vi "AB_API Add Source Item To Array.vi"(8 "error in (no error)":errorcluster, 9 "source item ID":string, 10 "buildObject":T1, 11 "source items in":refnum<class "AB_Source.lvclass">[](array[class])) -> (0 "error out":errorcluster, 1 "index":i32, 2 "added?":bool, 3 "source items out":refnum<class "AB_Source.lvclass">[](array[class]))   [LabVIEW 2020]
uses:
  <vilib>/AppBuilder/AB_Classes/Source/AB_Source.lvclass
  <resource>/Framework/Providers/API/ItemRef.ctl
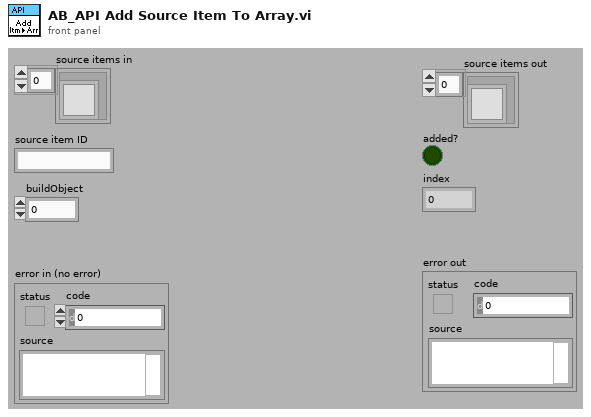
[diagram p1: front panel]
types:
  T1 = typedef "ItemRef.ctl" = u64
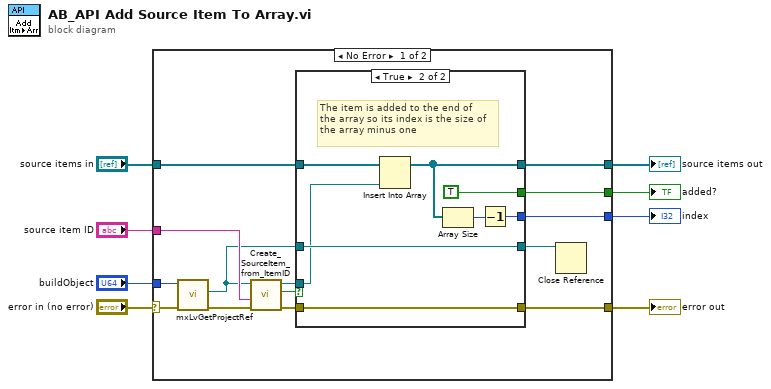
[diagram p0: block diagram]
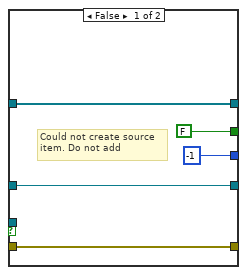
[diagram p2: hidden frame]
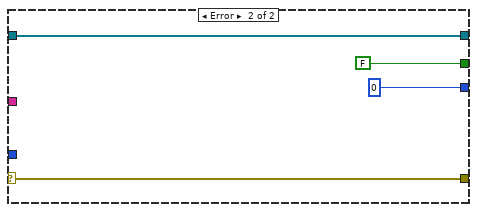
[diagram p3: hidden frame]
diagram:
  n1 = case shown="No Error" "error in (no error)" {
    selector: "error in (no error)" -> [w13 w39]
    tunnel: "source item ID" -> [w18 _]
    tunnel: [w12 w39] -> w7
    tunnel: [w17 0] -> w6
    tunnel: [w9 w38] -> w5
    tunnel: [w16 FALSE] -> w4
    tunnel: "source items in" -> [w15 w38]
    tunnel: "buildObject" -> [w14 _]
    frame No Error {
      n2 = call <resource>:"mxLvGetProjectRef.vi"("error in"=w13, "Item"=w14) -> ("error out"=w20:errorcluster, "Project Refnum"=w11:refnum<vi>)  [unwired: 8 out]
      n3 = call <vilib>:"Create_SourceItem_from_ItemID.vi"("error in (no error)"=w20, "itemID"=w18, "Project Refnum"=w11) -> ("error out"=w22:errorcluster, "valid?"=w19:bool, "AB_Source out"=w21:refnum<class "AB_Source.lvclass">)  [unwired: 6 in]
      n4 = case shown="True" w19 {
        tunnel: w22 -> [w25 w29]
        tunnel: [w25 w29] -> w12
        tunnel: w21 -> [_ w28]
        tunnel: [w24 w31] -> w9
        tunnel: w15 -> [w24 w32]
        tunnel: [-1 w33] -> w17
        tunnel: [FALSE TRUE] -> w16
        tunnel: w11 -> [w23 w30]
        tunnel: [w23 w30] -> w10
        frame False {
          # "Could not create source\nitem. Do not add"
        }
        frame True {
          # "The item is added to the end of\nthe array so its index is the size of \nthe array minus one"
          n5 = Insert Into Array(array=w32, new element=w28) -> (w31:refnum<class "AB_Source.lvclass">[])  [unwired: 1 in]
          n6 = Array Size(array=w31) -> (size(s)=w34:i32)
          n7 = Decrement(x=w34) -> (x-1=w33:i32)
        }
      }
      n8 = Close Reference(reference=w10) -> ()  [unwired: 1 in, 1 out]
    }
    frame Error {
    }
  }
  "error out" <- w7
  "index" <- w6
  "source items out" <- w5
  "added?" <- w4
